vi "Find Angle to Goal.vi"(7 "rollover?":bool=TRUE, 8 "Goal Column":i32, 9 "Goal Row":i32, 10 "Column":i32, 11 "Row":i32) -> (0 "goal column out":i32, 1 "goal row out":i32, 2 "distance":dbl, 3 "angle (deg)":dbl)   [LabVIEW 2017, in "DS Square.lvlib"]
uses:
  DS Square.lvlib
  SubVIs/Read-Only Globals.vi
  SubVIs/Globals (private).vi
  Square/Square.lvclass
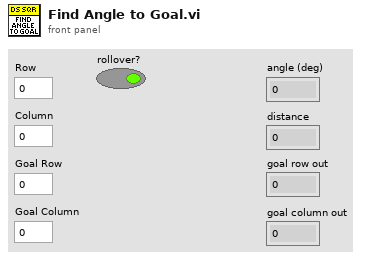
[diagram p1: front panel]
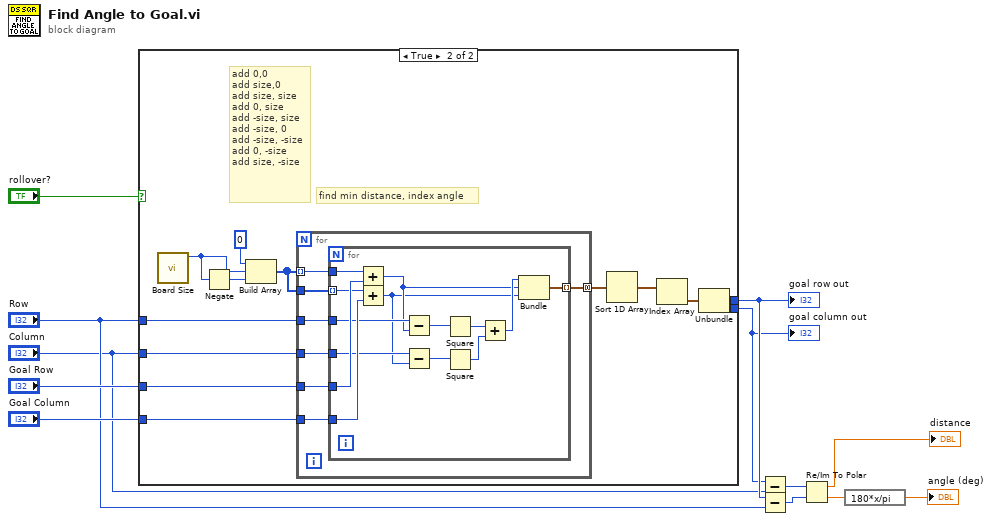
[diagram p0: block diagram]
diagram:
  n1 = case shown="True" "rollover?" {
    tunnel: "Goal Row" -> [w14 w23]
    tunnel: "Goal Column" -> [w13 w22]
    tunnel: "Row" -> [_ w18]
    tunnel: [w14 w17] -> w8
    tunnel: "Column" -> [_ w16]
    tunnel: [w13 w15] -> w2
    frame False {
    }
    frame True {
      # "find min distance, index angle"
      # "add 0,0\nadd size,0\nadd size, size\nadd 0, size\nadd -size, size\nadd -size, 0\nadd -size, -size\nadd 0, -size\nadd size, -size"
      n2 = call "Board Size.vi"() -> ("Board Size"=w27:i32)  [unwired: 11 in]
      n3 = Negate(x=w27) -> (-x=w26:i32)
      n4 = Build Array(0 ("element"), w27, w26) -> (w24:i32[])
      n5 = for {
        tunnel: w24 -> [w34] mode=indexing
        tunnel: w24 -> [w33]
        tunnel: w18 -> [w32]
        tunnel: w16 -> [w31]
        tunnel: w23 -> [w30]
        tunnel: w22 -> [w29]
        tunnel: [w28] -> w21 mode=concatenating
        n6 = for {
          tunnel: w34 -> [w48]
          tunnel: w33 -> [w46] mode=indexing
          tunnel: w32 -> [w44]
          tunnel: w31 -> [w43]
          tunnel: w30 -> [w47]
          tunnel: w29 -> [w45]
          tunnel: [w39] -> w28 mode=indexing
          n7 = Add(x=w48, y=w47) -> (x+y=w36:i32)
          n8 = Add(x=w46, y=w45) -> (x+y=w35:i32)
          n9 = Subtract(x=w44, y=w36) -> (x-y=w38:i32)
          n10 = Subtract(x=w43, y=w35) -> (x-y=w37:i32)
          n11 = Square(x=w38) -> (x^2=w42:i32)
          n12 = Square(x=w37) -> (x^2=w41:i32)
          n13 = Add(x=w42, y=w41) -> (x+y=w40:i32)
          n14 = Bundle(w40, w36, w35) -> (w39:cluster{i32, i32, i32})  [unwired: 1 in]
        }
      }
      n15 = Sort 1D Array(array=w21) -> (sorted array=w20:cluster{i32, i32, i32}[])
      n16 = Index Array(array=w20) -> (element=w19:cluster{i32, i32, i32})  [unwired: 1 in]
      n17 = Unbundle(w19) -> (w17:i32, w15:i32)  [unwired: 1 out]
    }
  }
  "goal row out" <- w8
  "goal column out" <- w2
  n18 = Subtract(x=w2, y="Column") -> (x-y=w6:i32)
  n19 = Subtract(x=w8, y="Row") -> (x-y=w5:i32)
  n20 = Re/Im To Polar(2:w5, 3:w6) -> (0:w4:dbl, 1:→"distance":dbl)
  n21 = expression code="180*x/pi"(w4) -> (→"angle (deg)":dbl)
